vi "S2C_Access_GetRefs.vi"(8 "Error In":errorcluster, 11 "VI Ref":refnum<vi>) -> (0 "Error Out":errorcluster)   [LabVIEW 2015]
doc: "Aquires a reference to key front panel controls and stores the reference in a global."
uses:
  S2C_Access_Globals.vi
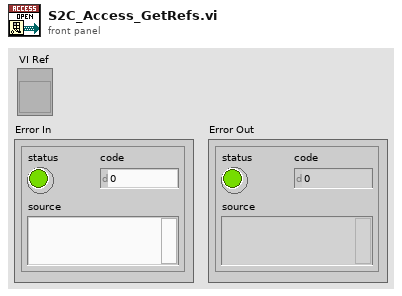
[diagram p1: front panel]
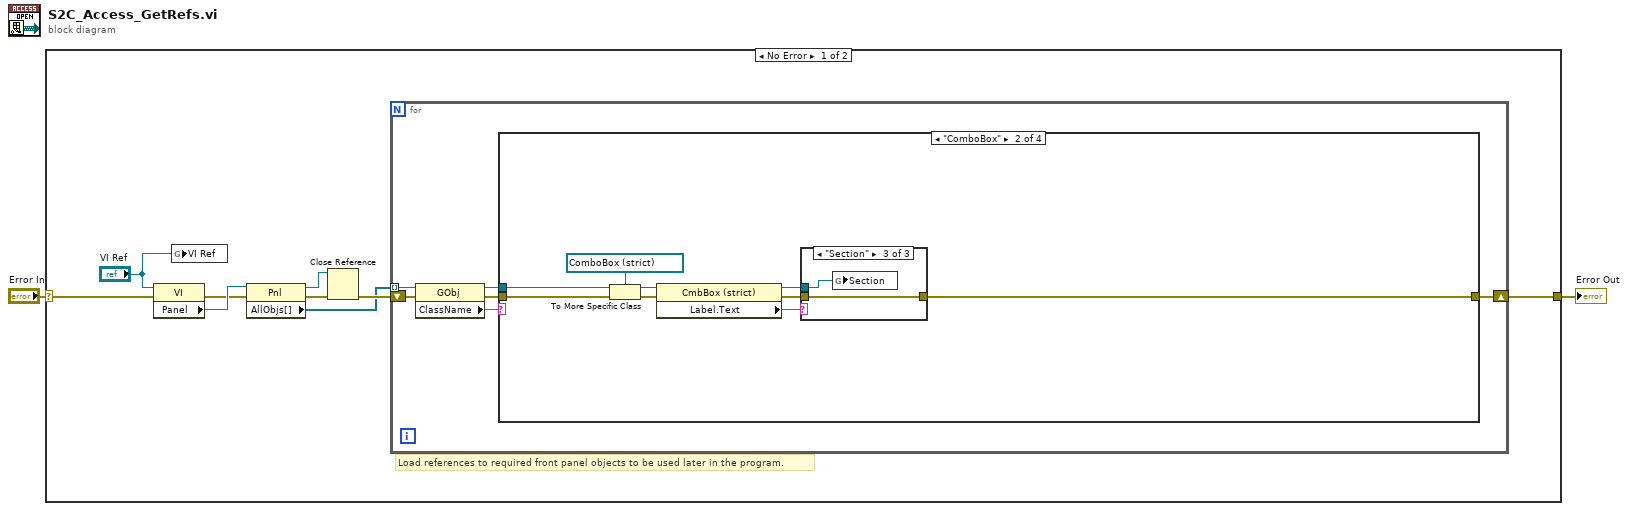
[diagram p0: block diagram]
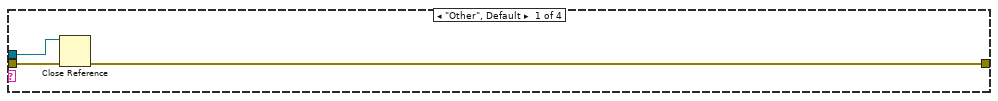
[diagram p2: hidden frame]
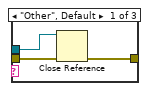
[diagram p3: hidden frame]
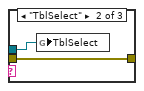
[diagram p4: hidden frame]
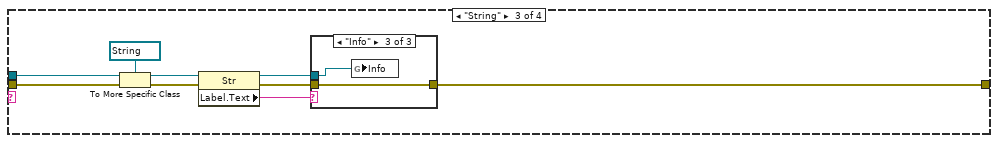
[diagram p5: hidden frame]
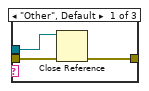
[diagram p6: hidden frame]
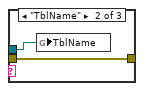
[diagram p7: hidden frame]
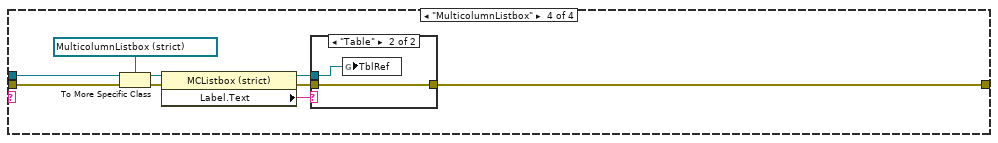
[diagram p8: hidden frame]
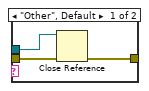
[diagram p9: hidden frame]
diagram:
  n1 = case shown="No Error" "Error In" {
    selector: "Error In" -> [w11 w67]
    tunnel: [w6 w67] -> w2
    frame No Error {
      # "Load references to required front panel objects to be used later in the program."
      n2 = property class="VI"(reference="VI Ref", error in=w11) -> (error out=w4:errorcluster, "Panel"=w5:refnum<vi>)  [unwired: 1 out]
      n3 = global write "S2C_Access_Globals.vi" "VI Ref"("VI Ref") -> ()
      n4 = property class="Pnl"(reference=w5, error in=w4) -> (reference out=w9:refnum<vi>, error out=w10:errorcluster, "AllObjs[]"=w7:refnum<vi>[])
      n5 = Close Reference(reference=w9, error in (no error)=w10) -> (error out=w8:errorcluster)
      n6 = for {
        shift-right: [w12] -> w6
        shift-left: w8 -> [w16]
        tunnel: w7 -> [w17] mode=indexing
        n7 = property class="GObj"(reference=w17, error in=w16) -> (reference out=w13:refnum<vi>, error out=w15:errorcluster, "ClassName"=w14:string)
        n8 = case shown="\"ComboBox\"" w14 {
          tunnel: w15 -> [w20 w23 w39 w55]
          tunnel: w13 -> [w19 w22 w38 w54]
          tunnel: [w18 w29 w45 w61] -> w12
          frame "Other", Default {
            n9 = Close Reference(reference=w19, error in (no error)=w20) -> (error out=w18:errorcluster)
          }
          frame "ComboBox" {
            n10 = To More Specific Class(target class=refnum<vi> refnum ("TblSelect"), reference=w22, error in=w23) -> (specific class reference=w27:refnum<vi>, error out=w28:errorcluster)
            n11 = property class="CmbBox (strict)"(reference=w27, error in=w28) -> (reference out=w24:refnum<vi>, error out=w25:errorcluster, "Label.Text"=w26:string)
            n12 = case shown="\"Section\"" w26 {
              tunnel: w25 -> [w32 w34 w36]
              tunnel: w24 -> [w30 w33 w35]
              tunnel: [w31 w34 w36] -> w29
              frame "Other", Default {
                n13 = Close Reference(reference=w30, error in (no error)=w32) -> (error out=w31:errorcluster)
              }
              frame "TblSelect" {
                n14 = global write "S2C_Access_Globals.vi" "TblSelect"(w33) -> ()
              }
              frame "Section" {
                n15 = global write "S2C_Access_Globals.vi" "Section"(w35) -> ()
              }
            }
          }
          frame "String" {
            n16 = To More Specific Class(target class=refnum<vi> refnum ("TblSelect"), reference=w38, error in=w39) -> (specific class reference=w43:refnum<vi>, error out=w44:errorcluster)
            n17 = property class="Str"(reference=w43, error in=w44) -> (reference out=w40:refnum<vi>, error out=w41:errorcluster, "Label.Text"=w42:string)
            n18 = case shown="\"Info\"" w42 {
              tunnel: w41 -> [w48 w50 w52]
              tunnel: w40 -> [w46 w49 w51]
              tunnel: [w47 w50 w52] -> w45
              frame "Other", Default {
                n19 = Close Reference(reference=w46, error in (no error)=w48) -> (error out=w47:errorcluster)
              }
              frame "TblName" {
                n20 = global write "S2C_Access_Globals.vi" "TblName"(w49) -> ()
              }
              frame "Info" {
                n21 = global write "S2C_Access_Globals.vi" "Info"(w51) -> ()
              }
            }
          }
          frame "MulticolumnListbox" {
            n22 = To More Specific Class(target class=refnum<vi> refnum ("TblRef"), reference=w54, error in=w55) -> (specific class reference=w59:refnum<vi>, error out=w60:errorcluster)
            n23 = property class="MCListbox (strict)"(reference=w59, error in=w60) -> (reference out=w56:refnum<vi>, error out=w57:errorcluster, "Label.Text"=w58:string)
            n24 = case shown="\"Table\"" w58 {
              tunnel: w57 -> [w64 w66]
              tunnel: w56 -> [w62 w65]
              tunnel: [w63 w66] -> w61
              frame "Other", Default {
                n25 = Close Reference(reference=w62, error in (no error)=w64) -> (error out=w63:errorcluster)
              }
              frame "Table" {
                n26 = global write "S2C_Access_Globals.vi" "TblRef"(w65) -> ()
              }
            }
          }
        }
      }
    }
    frame Error {
    }
  }
  "Error Out" <- w2
